vi "RP100.Get Output State.vi"(8 "error in (no error)":errorcluster, 10 "Output Channel":T1, 11 "VISA resource name":refnum<visa-resource-name>) -> (0 "error out":errorcluster, 1 "Output State":T2=enum."Enabled", 2 "Output Channel":T1, 3 "VISA Refnum out":refnum<visa-resource-name>)   [LabVIEW 2019, in "RP100.lvclass"]
uses:
  RP100.lvclass
  4adffc19-9644-49fa-a49d-0b54b09e0f06.vi
  Typedefs/Output Channel--Enum.ctl
  Typedefs/Output State--Enum.ctl
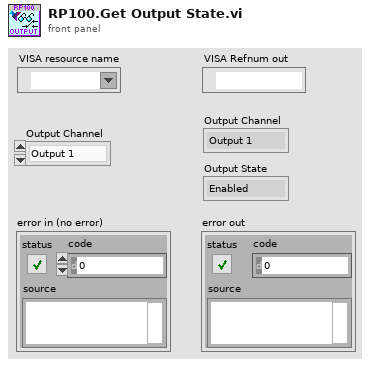
[diagram p1: front panel]
types:
  T1 = typedef "RP100.lvclass/Output Channel--Enum.ctl" = enum16{"Output 1", "Output 2"}
  T2 = typedef "RP100.lvclass/Output State--Enum.ctl" = enum16{"Shorted", "Enabled"}
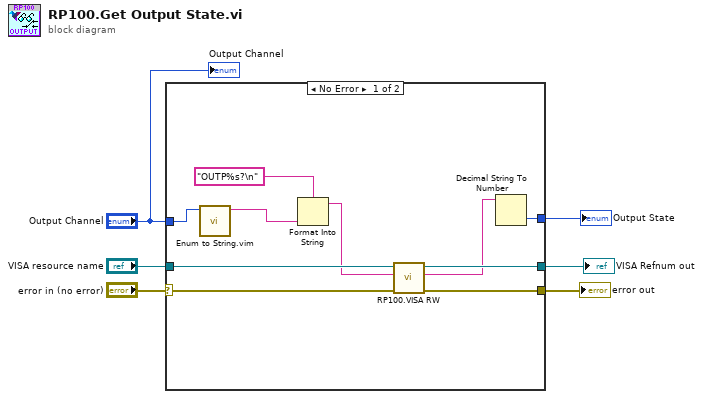
[diagram p0: block diagram]
diagram:
  n1 = case shown="No Error" "error in (no error)" {
    selector: "error in (no error)" -> [w12 w18]
    tunnel: "VISA resource name" -> [w11 w17]
    tunnel: "Output Channel" -> [w14 _]
    tunnel: [w9 w17] -> w5
    tunnel: [w16 _] -> w4
    tunnel: [w7 w18] -> w3
    frame No Error {
      n2 = call "Enum to String.vim"("Command"=w14) -> ("Command"=w15:string)  [unwired: 9 in, 1 out]
      n3 = Format Into String(format string="OUTP%s?\n", w15) -> (resulting string=w10:string)  [unwired: 2 in, 1 out]
      n4 = call "RP100.VISA RW.vi"("error in (no error)"=w12, "Write"=w10, "VISA Refnum in"=w11) -> ("error out"=w7:errorcluster, "Read"=w8:string, "VISA Refnum out"=w9:refnum<visa-resource-name>)  [unwired: 6 in]
      n5 = Decimal String To Number(string=w8) -> (number=w16:i32)  [unwired: 2 in, 1 out]
    }
    frame Error {
    }
  }
  "VISA Refnum out" <- w5
  "error out" <- w3
  "Output State" <- w4
  "Output Channel" <- "Output Channel"
